vi "SetLevel.vi"(8 "error in (no error)":errorcluster, 10 "Level (dBm)":dbl, 11 "PwrMtr_U2k in":refnum<class "PwrMtr_U2k.lvclass">) -> (0 "error out":errorcluster, 3 "PwrMtr_U2k out":refnum<class "PwrMtr_U2k.lvclass">)   [LabVIEW 2014, in "PwrMtr_U2k.lvclass"]
uses:
  PwrMtr_U2k.lvclass
  PwrMtr_U2k.lvclass/PwrMtr_U2k.ctl
  data/Agilent U2000 Series.lvlib
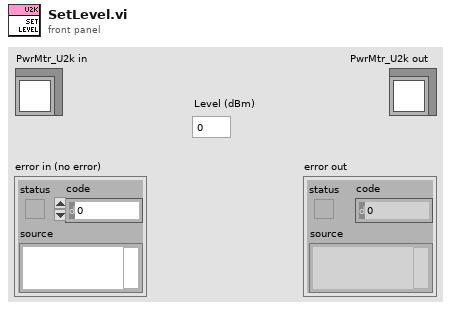
[diagram p1: front panel]
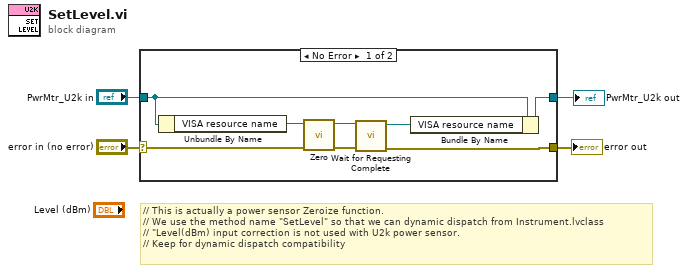
[diagram p0: block diagram]
diagram:
  # "// This is actually a power sensor Zeroize function.\n// We use the method name \"SetLevel\" so that we can dynamic dispatch from Instrument.lvclass\n// \"Level(dBm) input correction is not used with U2k power sensor. \n// Keep for dynamic dispatch compatibility"
  n1 = case shown="No Error" "error in (no error)" {
    selector: "error in (no error)" -> [w10 w14]
    tunnel: "PwrMtr_U2k in" -> [w12 w13]
    tunnel: [w11 w13] -> w3
    tunnel: [w9 w14] -> w1
    frame No Error {
      n2 = Unbundle By Name(w12) -> ("VISA resource name"=w8:refnum<visa-resource-name>)
      n3 = call "Zero.vi"("error in (no error)"=w10, "VISA resource name"=w8) -> ("error out"=w7:errorcluster, "VISA resource name out"=w6:refnum<visa-resource-name>)  [unwired: 8 in]
      n4 = call "Wait for Requesting Complete.vi"("error in (no error)"=w7, "VISA resource name"=w6) -> ("error out"=w9:errorcluster, "VISA resource name out"=w5:refnum<visa-resource-name>)  [unwired: 8 in]
      n5 = Bundle By Name(cluster=w12, "VISA resource name"=w5) -> (w11:refnum<class "PwrMtr_U2k.lvclass">)
    }
    frame Error {
    }
  }
  "error out" <- w1
  "PwrMtr_U2k out" <- w3
